vi "Poll Web Variables For Changes.vi"(8 "error in (no error)":errorcluster, 11 "Queue in":refnum<queue>) -> ()   [LabVIEW 2014]
uses:
  controls/UI DataSam.ctl
  controls/Variables to check enum.ctl
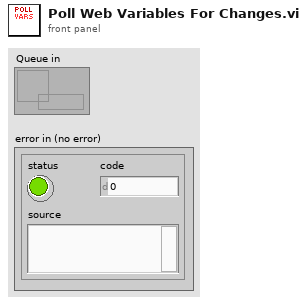
[diagram p1: front panel]
types:
  T1 = typedef "Variables to check enum.ctl" = enum16{"Connect", "Control", "Direction"}
  T2 = typedef "UI DataSam.ctl" = cluster{"Message":string, "Data":variant}
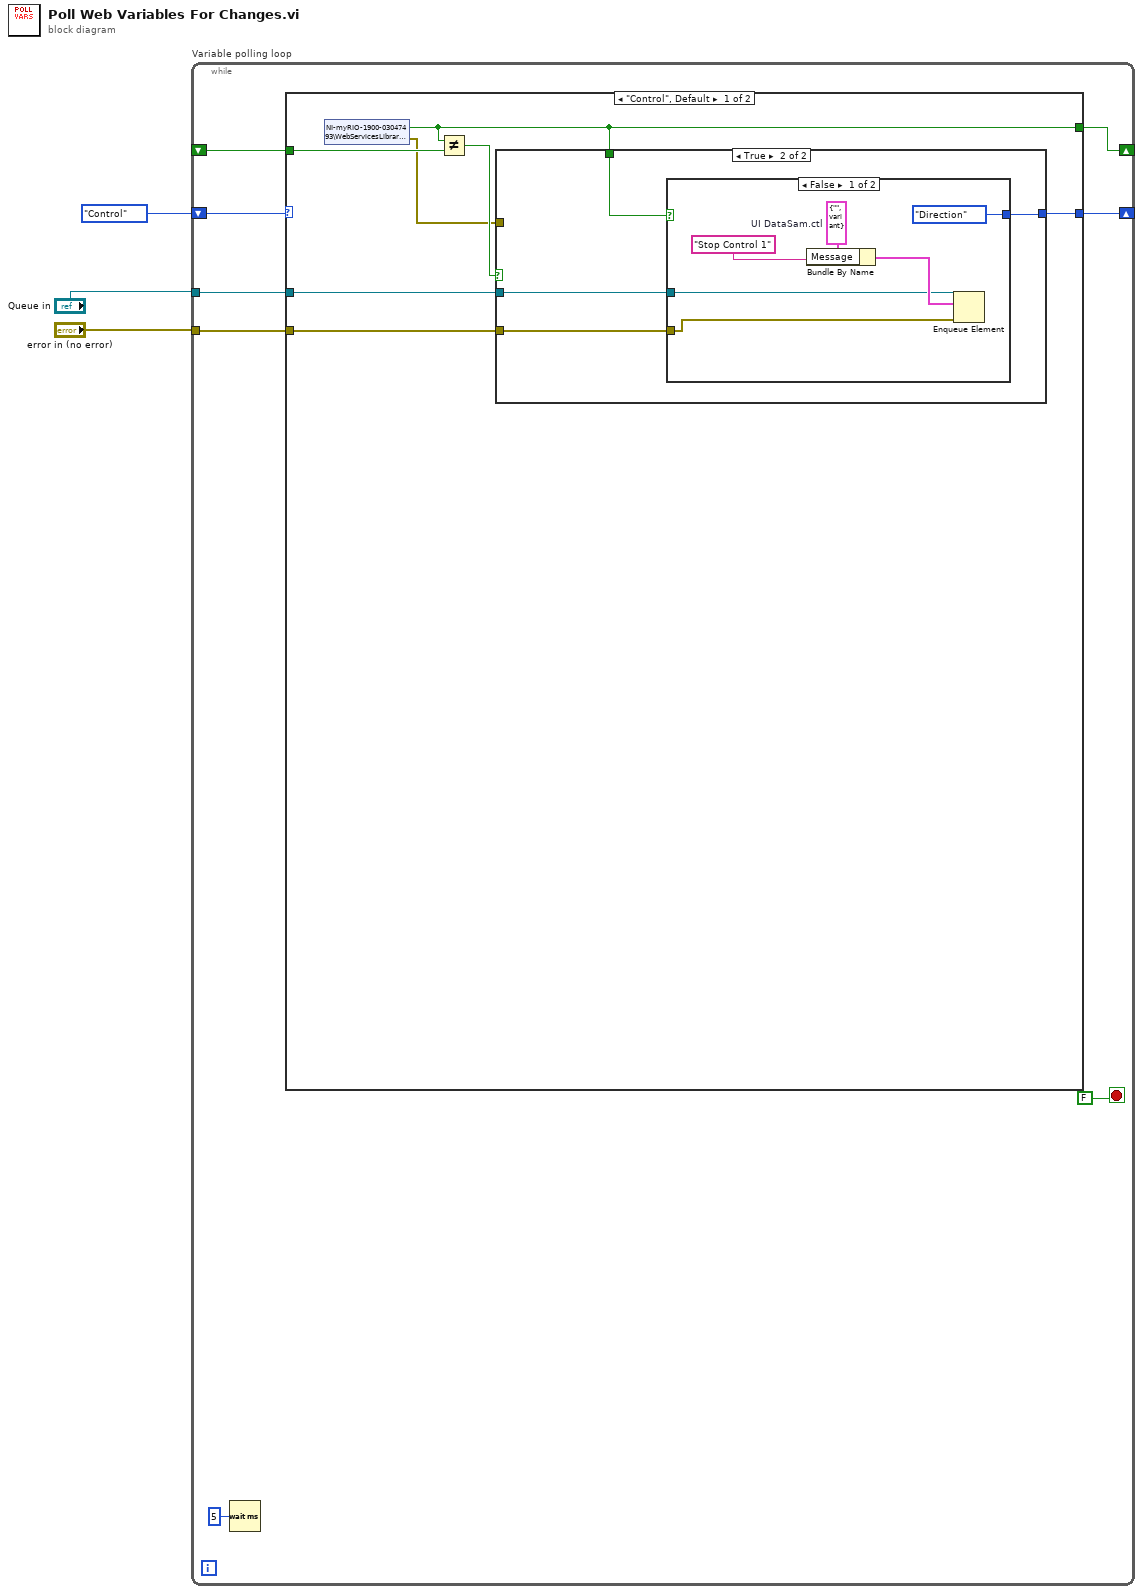
[diagram p0: block diagram]
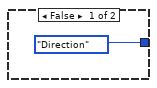
[diagram p2: hidden frame]
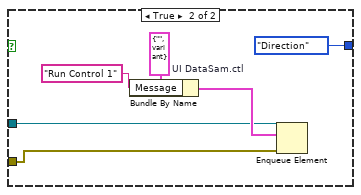
[diagram p3: hidden frame]
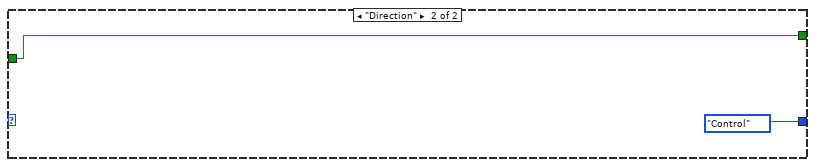
[diagram p4: hidden frame]
diagram:
  n1 = while "Variable polling loop" {
    tunnel: "Queue in" -> [w11]
    tunnel: "error in (no error)" -> [w10]
    shift-right: [w6] -> _
    shift-left: Variables_to_check_enum."Control" ("Command Parser Enum") -> [w9]
    shift-right: [w7] -> _
    shift-left: _ -> [w8]
    stop <- FALSE stop-if-true
    n2 = Wait (ms)(milliseconds to wait=u32 5) -> ()  [unwired: 1 out]
    n3 = case shown="\"Control\", Default" w9 {
      tunnel: w11 -> [w15 _]
      tunnel: w10 -> [w14 _]
      tunnel: w8 -> [w17 w36]
      tunnel: [w12 w36] -> w7
      tunnel: [w13 Variables_to_check_enum."Control" ("Command Parser Enum")] -> w6
      frame "Control", Default {
        n4 = shared-variable "NI-myRIO-1900-03047493\\WebServicesLibrary.lvlib\\Control"() -> (w12:bool, error out=w16:errorcluster)  [unwired: 1 in]
        n5 = Not Equal?(x=w12, y=w17) -> (x != y?=w18:bool)
        n6 = case shown="True" w18 {
          tunnel: w16 -> [_ _]
          tunnel: w15 -> [_ w23]
          tunnel: w14 -> [_ w22]
          tunnel: [Variables_to_check_enum."Direction" ("Command Parser Enum") w21] -> w13
          tunnel: w12 -> [_ w20]
          frame False {
          }
          frame True {
            n7 = case shown="False" w20 {
              tunnel: w23 -> [w26 w32]
              tunnel: w22 -> [w25 w31]
              tunnel: [Variables_to_check_enum."Direction" ("Command Parser Enum") Variables_to_check_enum."Direction" ("Command Parser Enum")] -> w21
              frame False {
                w27 = T2 {"Message"="", "Data"=variant}  # UI DataSam.ctl
                n8 = Bundle By Name(cluster=w27, "Message"="Stop Control 1") -> (w28:T2)
                n9 = Enqueue Element(queue=w26, element=w28, error in (no error)=w25) -> ()  [unwired: 1 in, 3 out]
              }
              frame True {
                w33 = T2 {"Message"="", "Data"=variant}  # UI DataSam.ctl
                n10 = Bundle By Name(cluster=w33, "Message"="Run Control 1") -> (w34:T2)
                n11 = Enqueue Element(queue=w32, element=w34, error in (no error)=w31) -> ()  [unwired: 1 in, 3 out]
              }
            }
          }
        }
      }
      frame "Direction" {
      }
    }
  }
